vi "DAQ_channel_setup.vi"(11 "Text Ring":enum16{"Test setup", "Microscope"}(ring)) -> (3 "DAQ channels OUT":T1={"CO.Pulse.Term"="/Dev2/PFI0", "Voice coil analog output"="Dev2/ao1", "counter"="Dev2/ctr1", "CO.Pulse.Term 2"="/Dev2/PFI1", "AOTF lines"="Dev2/port0/line0:3", "counter 2"="Dev2/ctr2", "CO.Pulse.Term 3"="/Dev2/PFI2", "counter 3"="Dev2/ctr1"})   [LabVIEW 2020]
uses:
  Calibration files/DAQ_channel_typedef.ctl
panel:
  in  "DAQ channels Microscope":T1={"CO.Pulse.Term"="/Dev1/PFI0", "Voice coil analog output"="Dev1/ao0", "counter"="Dev1/ctr0", "CO.Pulse.Term 2"="/Dev1/PFI12", "AOTF lines"="Dev1/port0/line24:23, Dev1/port0/line20:19", "counter 2"="Dev1/ctr1", "CO.Pulse.Term 3"="/Dev1/PFI14", "counter 3"="Dev1/ctr2"}
  in  "DAQ channels Test setup":T1={"CO.Pulse.Term"="/Dev2/PFI0", "Voice coil analog output"="Dev2/ao1", "counter"="Dev2/ctr0", "CO.Pulse.Term 2"="/Dev2/PFI1", "AOTF lines"="Dev2/port0/line0:3", "counter 2"="Dev2/ctr1", "CO.Pulse.Term 3"="/Dev2/PFI2", "counter 3"="Dev2/ctr2"}
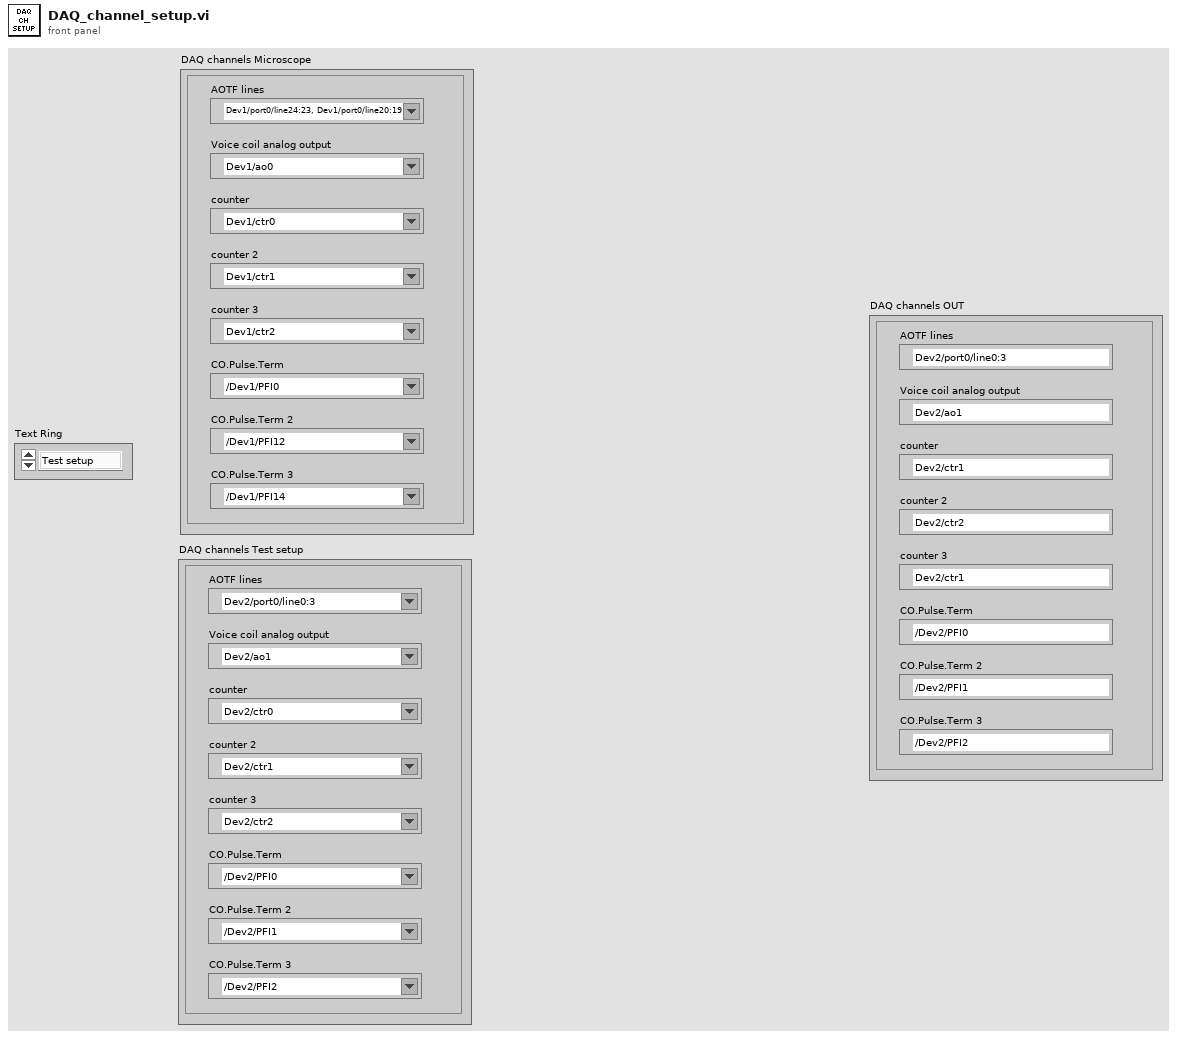
[diagram p1: front panel]
types:
  T1 = typedef "DAQ_channel_typedef.ctl" = cluster{"CO.Pulse.Term":tag, "Voice coil analog output":tag, "counter":tag, "CO.Pulse.Term 2":tag, "AOTF lines":tag, "counter 2":tag, "CO.Pulse.Term 3":tag, "counter 3":tag}
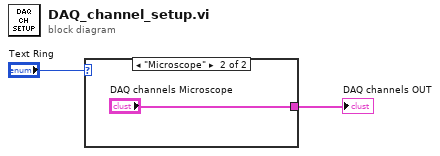
[diagram p0: block diagram]
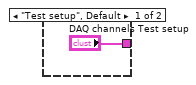
[diagram p2: hidden frame]
diagram:
  n1 = case shown="\"Microscope\"" "Text Ring" {
    tunnel: ["DAQ channels Test setup" "DAQ channels Microscope"] -> w1
    frame "Test setup", Default {
    }
    frame "Microscope" {
    }
  }
  "DAQ channels OUT" <- w1
